vi "Calculate Dilution.vi"(8 "error in (no error)":errorcluster, 11 "cRIO-CO2 in":refnum<class "cRIO-CO2.lvclass">) -> (0 "error out":errorcluster, 1 "Dilute":bool, 2 "He mBar":dbl, 3 "cRIO-CO2 out":refnum<class "cRIO-CO2.lvclass">)   [LabVIEW 2015, in "cRIO-Carbondioxide.lvlib" / "cRIO-CO2.lvlib" / "cRIO-CO2.lvclass"]
uses:
  cRIO-CO2.lvclass
  cRIO-CO2.lvclass/cRIO-CO2.ctl
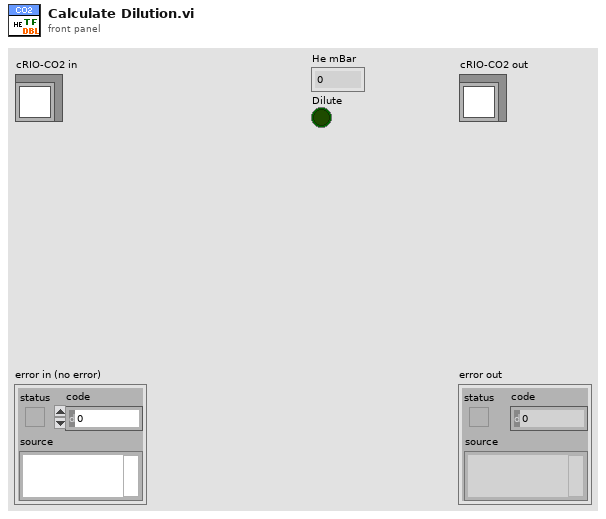
[diagram p1: front panel]
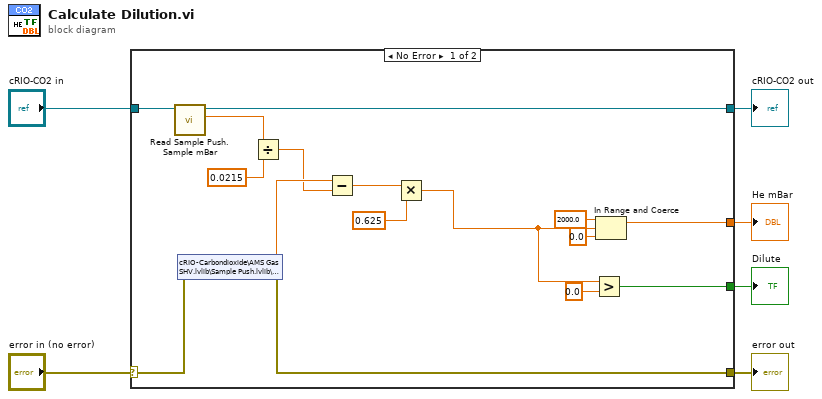
[diagram p0: block diagram]
diagram:
  n1 = case shown="No Error" "error in (no error)" {
    selector: "error in (no error)" -> [w20 w24]
    tunnel: [w19 w24] -> w5
    tunnel: [w21 w23] -> w3
    tunnel: "cRIO-CO2 in" -> [w22 w23]
    tunnel: [w18 _] -> w2
    tunnel: [w14 _] -> w1
    frame No Error {
      n2 = call "Read Sample Push.Sample mBar.vi"("cRIO-CO2 in"=w22) -> ("Sample mBar"=w13:dbl, "cRIO-CO2 out"=w21:refnum<class "cRIO-CO2.lvclass">)  [unwired: 9 in]
      n3 = shared-variable "cRIO-Carbondioxide\\AMS Gas SHV.lvlib\\Sample Push.lvlib\\Initial mBar"(error in=w20) -> (w11:dbl, error out=w19:errorcluster)
      n4 = Divide(x=w13, y=0.0215 ("a")) -> (x/y=w10:dbl)
      n5 = Subtract(x=w11, y=w10) -> (x-y=w9:dbl)
      n6 = Multiply(x=w9, y=0.625) -> (x*y=w7:dbl)
      n7 = Greater?(x=w7, y=0.0) -> (0:w14:bool)
      n8 = In Range and Coerce(upper limit=2000.0, x=w7, lower limit=0.0) -> (coerced(x)=w18:dbl)  [unwired: 1 out]
    }
    frame Error {
    }
  }
  "error out" <- w5
  "cRIO-CO2 out" <- w3
  "He mBar" <- w2
  "Dilute" <- w1
